vi "Process raw data.vi"(0 "reference in":refnum<class "Force Curve_tdms.lvclass">, 5 "error in (no error)":errorcluster) -> (14 "reference out":refnum<class "Force Curve_tdms.lvclass">, 19 "error out":errorcluster)   [LabVIEW 2019, in "Force Curve_tdms.lvclass"]
uses:
  Force Curve_tdms.lvclass
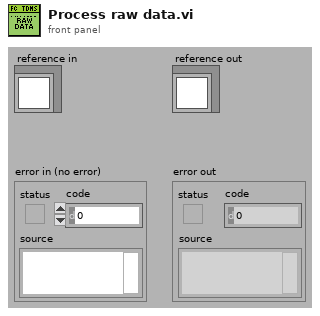
[diagram p1: front panel]
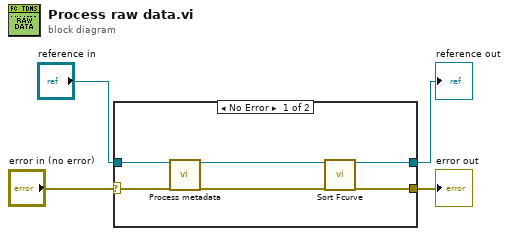
[diagram p0: block diagram]
diagram:
  n1 = case shown="No Error" "error in (no error)" {
    selector: "error in (no error)" -> [w9 w12]
    tunnel: [w5 w12] -> w3
    tunnel: [w7 w11] -> w1
    tunnel: "reference in" -> [w10 w11]
    frame No Error {
      n2 = call "Process metadata.vi"("reference in"=w10, "error in (no error)"=w9) -> ("reference out"=w6:refnum<class "Force Curve_tdms.lvclass">, "error out"=w8:errorcluster)  [unwired: 16 in]
      n3 = call "Sort Fcurve.vi"("reference in"=w6, "error in (no error)"=w8) -> ("reference out"=w7:refnum<class "Force Curve_tdms.lvclass">, "error out"=w5:errorcluster)  [unwired: 16 in]
    }
    frame Error {
    }
  }
  "error out" <- w3
  "reference out" <- w1
